vi "subCalcPropPageCtlName.vi"(1 "Property Page Ctl Label":string, 2 "Express VI Ctl Label":string) -> (0 "Prop Ctl Name":string)   [LabVIEW 2017]
doc: "Outputs the Property Page Ctl Label unless it is an empty string, then the Express VI Ctl Label is the output."
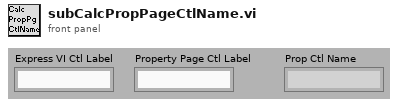
[diagram p1: front panel]
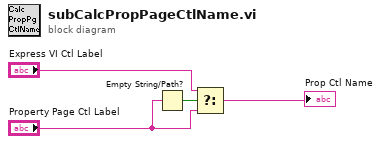
[diagram p0: block diagram]
diagram:
  n1 = Empty String/Path?(string/path="Property Page Ctl Label") -> (empty?=w2:bool)
  n2 = Select(t="Express VI Ctl Label", s=w2, f="Property Page Ctl Label") -> (s? t:f=→"Prop Ctl Name":string)
